vi "Set Plot Names.vi"(8 "에러 입력(에러 없음)":errorcluster, 10 "플롯 이름":string[](array[string]), 11 "그래프 참조":refnum<vi>) -> (0 "에러 출력":errorcluster)   [LabVIEW 2010]
doc: "웨이브폼 차트 또는 웨이브폼 그래프에서 플롯 이름을 설정하는데 이 VI를 사용합니다."
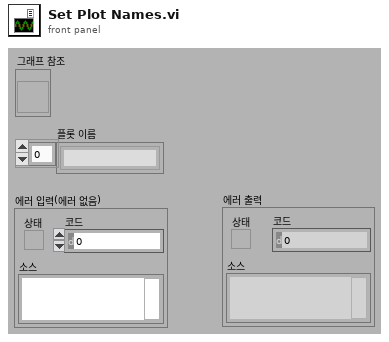
[diagram p1: front panel]
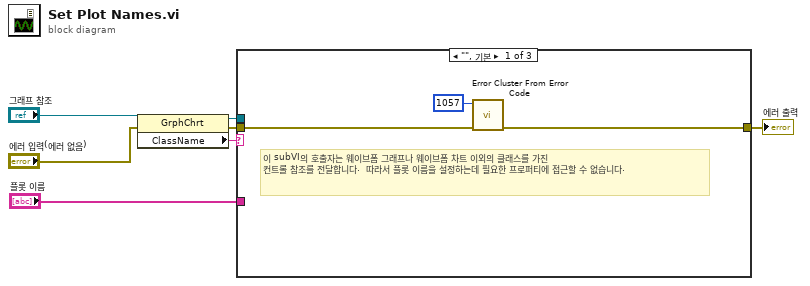
[diagram p0: block diagram]
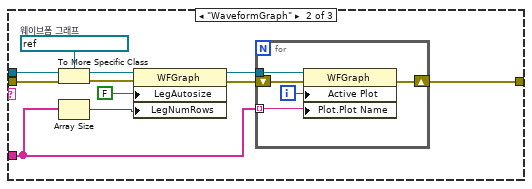
[diagram p2: hidden frame]
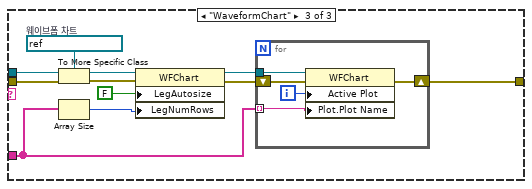
[diagram p3: hidden frame]
diagram:
  n1 = property class="GrphChrt"(reference="그래프 참조", error in="에러 입력(에러 없음)") -> (reference out=w4:refnum<vi>, error out=w5:errorcluster, "ClassName"=w6:string)
  n2 = case shown="\"\", 기본" w6 {
    tunnel: w5 -> [w9 w15 w31]
    tunnel: w4 -> [_ w16 w32]
    tunnel: "플롯 이름" -> [_ w11 w27]
    tunnel: [w8 w13 w29] -> w1
    frame "", Default {
      # "이 subVI의 호출자는 웨이브폼 그래프나 웨이브폼 차트 이외의 클래스를 가진 \n컨트롤 참조를 전달합니다.  따라서 플롯 이름을 설정하는데 필요한 프로퍼티에 접근할 수 없습니다."
      n3 = call <vilib>:"Error Cluster From Error Code.vi"("error in (no error)"=w9, "error code (0)"=1057) -> ("error out"=w8:errorcluster)  [unwired: 7 in]
    }
    frame "WaveformGraph" {
      w21 = refnum<vi> refnum  # 웨이브폼 그래프
      n4 = To More Specific Class(target class=w21, reference=w16, error in=w15) -> (specific class reference=w19:refnum<vi>, error out=w20:errorcluster)
      n5 = Array Size(array=w11) -> (size(s)=w12:i32)
      n6 = property class="WFGraph"(reference=w19, error in=w20, "LegAutosize"=FALSE ("Legend:Autosize"), "LegNumRows"=w12) -> (reference out=w17:refnum<vi>, error out=w14:errorcluster)
      n7 = for {
        tunnel: w17 -> [w26]
        shift-right: [w24] -> w13
        shift-left: w14 -> [w25]
        tunnel: w11 -> [w22] mode=indexing
        i -> [w23]
        n8 = property class="WFGraph"(reference=w26, error in=w25, "Active Plot"=w23, "Plot.Plot Name"=w22) -> (error out=w24:errorcluster)  [unwired: 1 out]
      }
    }
    frame "WaveformChart" {
      w37 = refnum<vi> refnum  # 웨이브폼 차트
      n9 = To More Specific Class(target class=w37, reference=w32, error in=w31) -> (specific class reference=w35:refnum<vi>, error out=w36:errorcluster)
      n10 = Array Size(array=w27) -> (size(s)=w28:i32)
      n11 = property class="WFChart"(reference=w35, error in=w36, "LegAutosize"=FALSE ("Legend:Autosize"), "LegNumRows"=w28) -> (reference out=w33:refnum<vi>, error out=w30:errorcluster)
      n12 = for {
        tunnel: w33 -> [w42]
        shift-right: [w40] -> w29
        shift-left: w30 -> [w41]
        tunnel: w27 -> [w38] mode=indexing
        i -> [w39]
        n13 = property class="WFChart"(reference=w42, error in=w41, "Active Plot"=w39, "Plot.Plot Name"=w38) -> (error out=w40:errorcluster)  [unwired: 1 out]
      }
    }
  }
  "에러 출력" <- w1
